vi "LaserMarked_IOPanel.vi"() -> ()   [LabVIEW 2019, in "MPC_Laser Marked.lvclass"]
uses:
  MPC_Laser Marked.lvclass
  Function/IO Folder/IO_VI/IOCtrl/Ctrl/IO Card_Type.ctl
  Function/IO Folder/IO_Class/IOCard.lvclass
  Function/IO Folder/IO_Class/IOCard.lvclass/IOCard.ctl
panel:
  in  "Tab Control":enum32{"Page 1", "Page 2"}(tab)
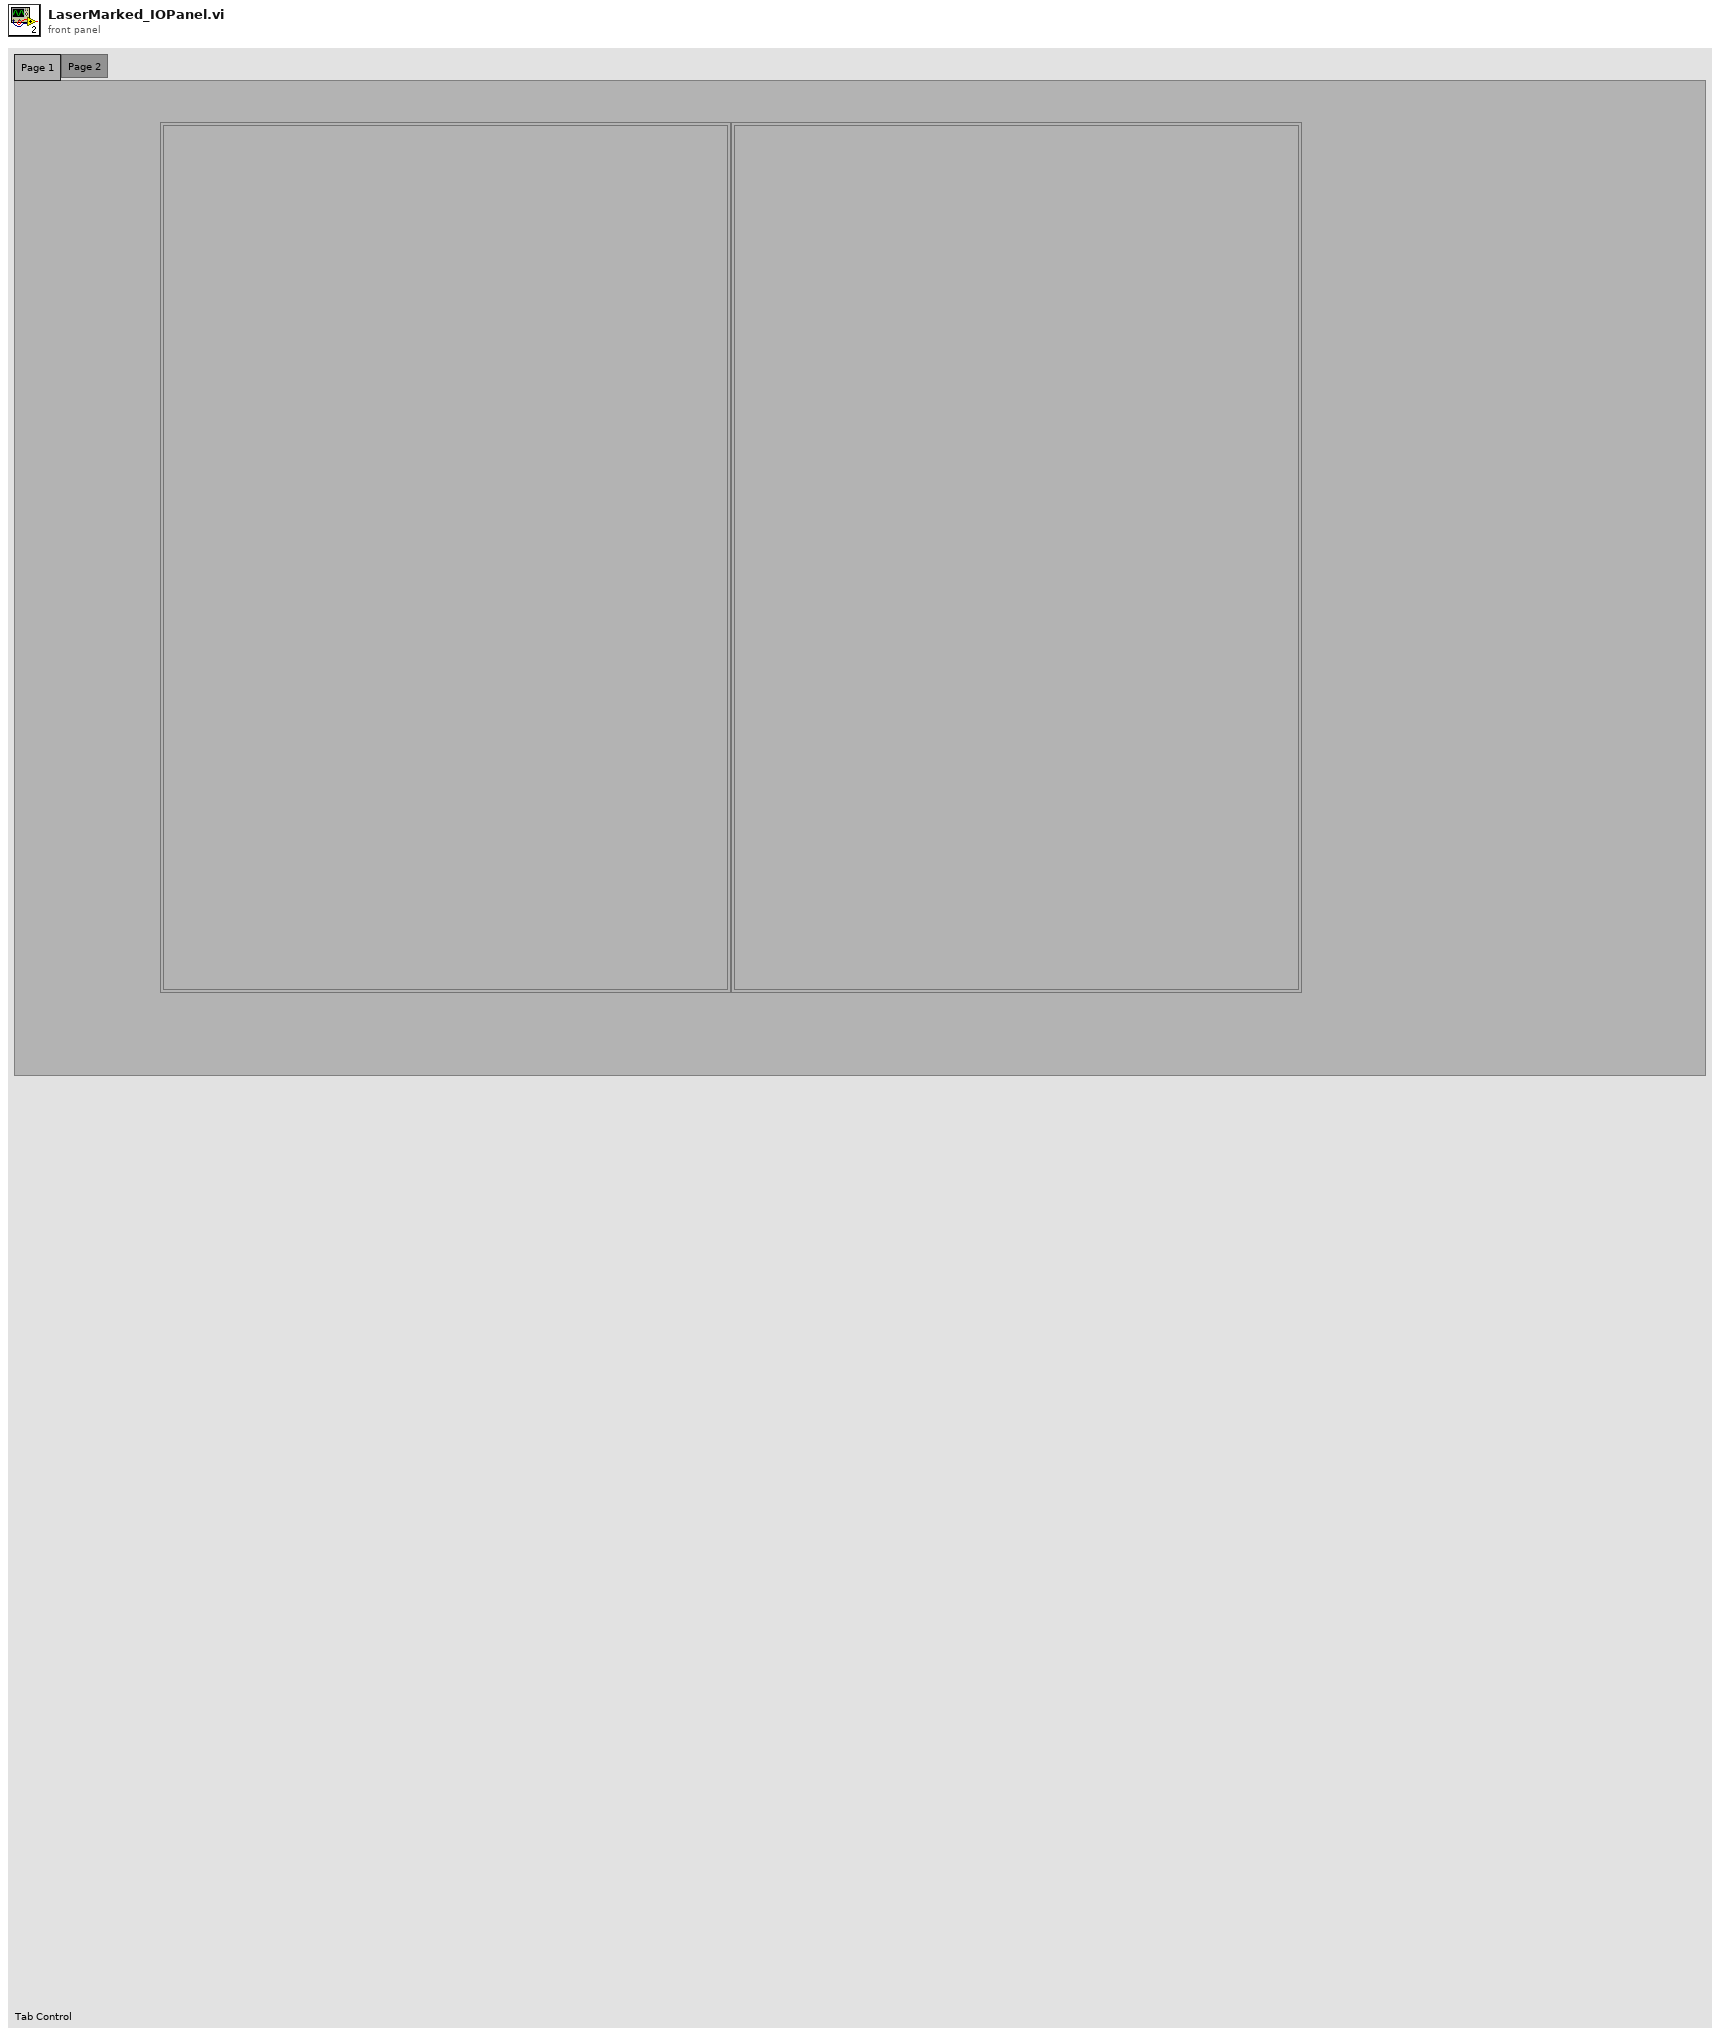
[diagram p1: front panel]
types:
  T1 = typedef "IO Card_Type.ctl" = enum16{"None", "Unidaq32", "6480", "2410C-64", "Zan", "DMC1000B", "16InOut", "Robot", "DMC3600"}
  T2 = cluster{"IO Card Type":T1, "IOType":enum16{"Input", "Output"}, "CardNumber":i32, "ConnectAct":bool, "IP":string}
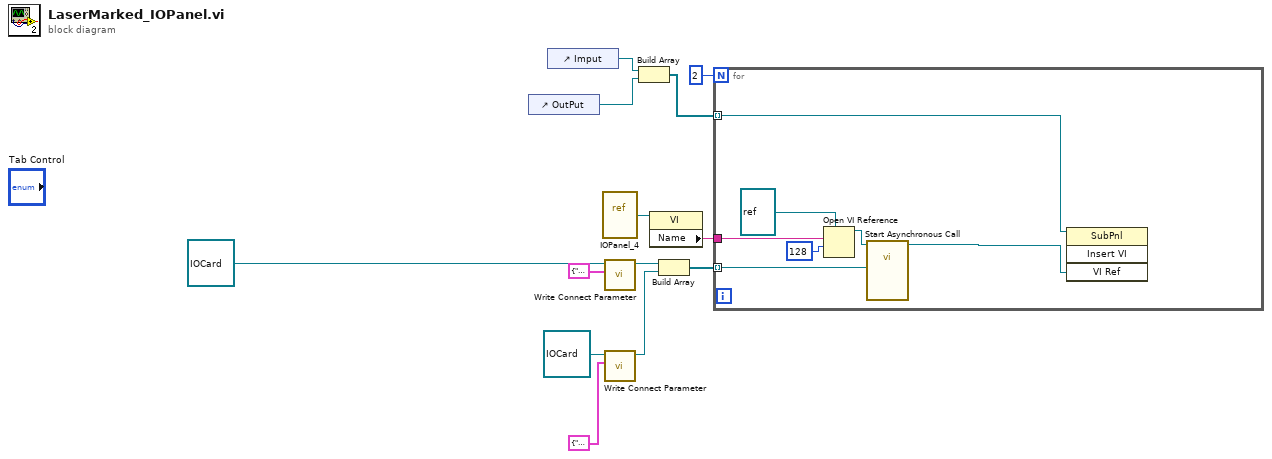
[diagram p0: block diagram]
diagram:
  n1 = control-ref of="OutPut"() -> (w2:refnum<vi>)
  n2 = control-ref of="Imput"() -> (w3:refnum<vi>)
  n3 = vi-ref "IOPanel_4.vi"() -> (w9:refnum<vi>)
  n4 = call "Write Connect Parameter.vi"("Connect Parameter"=T2 {"IO Card Type"=enum."DMC1000B", "IOType"=enum."Input", "CardNumber"=0, "ConnectAct"=FALSE, "IP"=""}, "IOCard in"=refnum<class "IOCard.lvclass"> refnum ("IOCard.lvclass")) -> ("IOCard out"=w6:refnum<class "IOCard.lvclass">)  [unwired: 8 in, 1 out]
  n5 = call "Write Connect Parameter.vi"("Connect Parameter"=T2 {"IO Card Type"=enum."DMC1000B", "IOType"=enum."Output", "CardNumber"=0, "ConnectAct"=FALSE, "IP"=""}, "IOCard in"=refnum<class "IOCard.lvclass"> refnum ("IOCard.lvclass")) -> ("IOCard out"=w5:refnum<class "IOCard.lvclass">)  [unwired: 8 in, 1 out]
  n6 = Build Array(w3, w2) -> (w1:refnum<vi>[])
  n7 = property class="VI"(reference=w9) -> ("Name"=w8:string)  [unwired: 1 in, 2 out]
  n8 = Build Array(w6, w5) -> (w4:refnum<class "IOCard.lvclass">[])
  n9 = for {
    N: 2 -> [_]
    tunnel: w8 -> [w20]
    tunnel: w4 -> [w16] mode=indexing
    tunnel: w1 -> [w15] mode=indexing
    n10 = Open VI Reference(type specifier VI Refnum (for type only)=refnum<vi> refnum, vi path=w20, options=128) -> (vi reference=w17:refnum<vi>)  [unwired: 3 in, 1 out]
    n11 = call-by-ref "Start Asynchronous Call"(reference=w17, "IOCard In"=w16) -> (reference out=w14:refnum<vi>)  [unwired: 12 in, 1 out]
    n12 = invoke class="SubPnl" method="Insert VI"(reference=w15, "VI Ref"=w14) -> ()  [unwired: 2 in, 4 out]
  }
